vi "Polymorphic - Open Connection.vi"   [LabVIEW 2021]
doc: "Opens a connection to a DAQiFi device. The input string should specify either an IP address or a COM port."
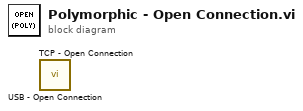
[diagram p0: block diagram]
diagram:
  n1 = call "USB - Open Connection.vi"() -> ()  [unwired: 10 in, 2 out]
  n2 = call "TCP - Open Connection.vi"() -> ()  [unwired: 10 in, 2 out]
